vi "Setup TS.vi"(8 "error in":errorcluster, 11 "HTS Test Stand in":refnum<class "HTS Test Stand.lvclass">) -> (0 "error out":errorcluster, 3 "HTS Test Stand out":refnum<class "HTS Test Stand.lvclass">)   [LabVIEW 2019, in "Test Stands.lvlib" / "HTS Test Stand.lvclass"]
uses:
  HTS Test Stand.lvclass
  C:/Users/wg/Documents/LV_Projects/test-stand/App/Generic Test Stand/Generic Test Stand.lvclass
  DAC/HTS/Vacum Valve/DAC Vacum Valve.lvclass
  C:/Users/wg/Documents/LV_Projects/test-stand/App/DAC/DAC.lvclass
  DAC/HTS/Vacum Pressure/DAC Vacum Pressure.lvclass
  DAC/HTS/DC Supply/DAC DC Supply.lvclass
  DAC/HTS/LN2 Temp/DAC LN2 Temp.lvclass
  DAC/HTS/HTS dU/DAC HTS dU.lvclass
  DAC/DAC.lvclass/DAC.ctl
  Generic Test Stand/Generic Test Stand.lvclass/Generic Test Stand.ctl
  Generic Test Stand/Generic Test Stand.lvclass
  DAC/DAC.lvclass
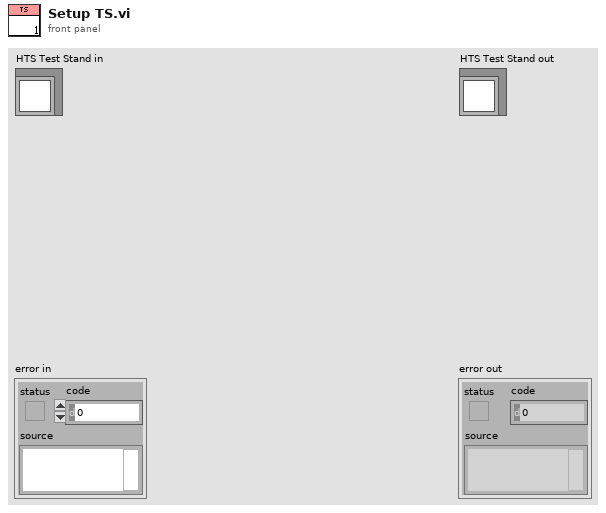
[diagram p1: front panel]
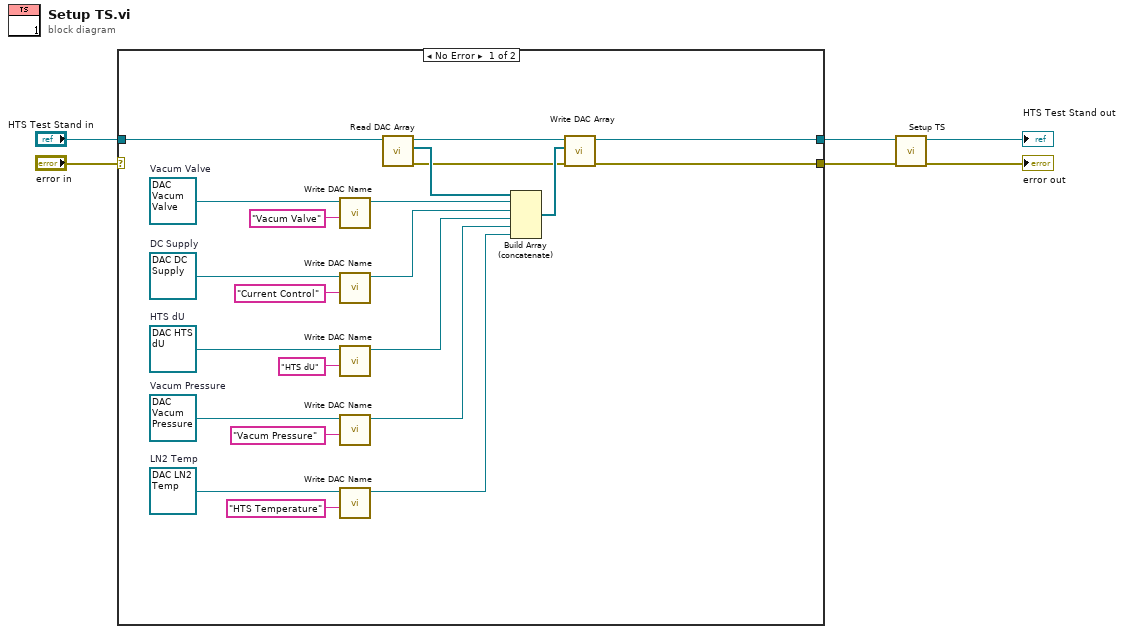
[diagram p0: block diagram]
diagram:
  n1 = case shown="No Error" "error in" {
    selector: "error in" -> [_ w29]
    tunnel: "HTS Test Stand in" -> [w28 w30]
    tunnel: [w22 w30] -> w2
    tunnel: [w21 w29] -> w1
    frame No Error {
      w11 = refnum<class "DAC HTS dU.lvclass"> refnum  # HTS dU
      w12 = refnum<class "DAC LN2 Temp.lvclass"> refnum  # LN2 Temp
      w13 = refnum<class "DAC DC Supply.lvclass"> refnum  # DC Supply
      w14 = refnum<class "DAC Vacum Pressure.lvclass"> refnum  # Vacum Pressure
      w15 = refnum<class "DAC Vacum Valve.lvclass"> refnum  # Vacum Valve
      n2 = call "Write DAC Name.vi"("DAC Name"="Vacum Valve", "DAC in"=w15) -> ("DAC out"=w23:refnum<class "DAC Vacum Valve.lvclass">)  [unwired: 8 in, 1 out]
      n3 = call "Write DAC Name.vi"("DAC Name"="Current Control", "DAC in"=w13) -> ("DAC out"=w10:refnum<class "DAC DC Supply.lvclass">)  [unwired: 8 in, 1 out]
      n4 = call "Write DAC Name.vi"("DAC Name"="HTS dU", "DAC in"=w11) -> ("DAC out"=w9:refnum<class "DAC HTS dU.lvclass">)  [unwired: 8 in, 1 out]
      n5 = call "Write DAC Name.vi"("DAC Name"="Vacum Pressure", "DAC in"=w14) -> ("DAC out"=w8:refnum<class "DAC Vacum Pressure.lvclass">)  [unwired: 8 in, 1 out]
      n6 = call "Write DAC Name.vi"("DAC Name"="HTS Temperature", "DAC in"=w12) -> ("DAC out"=w7:refnum<class "DAC LN2 Temp.lvclass">)  [unwired: 8 in, 1 out]
      n7 = call "Read DAC Array.vi"("Generic Test Stand in"=w28) -> ("error out"=w24:errorcluster, "DAC Array"=w27:refnum<class "DAC.lvclass">[], "Generic Test Stand out"=w26:refnum<class "HTS Test Stand.lvclass">)  [unwired: 8 in]
      n8 = Build Array (concatenate)(w27, w23, w10, w9, w8, w7) -> (w25:refnum<class "DAC.lvclass">[])
      n9 = call "Write DAC Array.vi"("error in (no error)"=w24, "DAC Array"=w25, "Generic Test Stand in"=w26) -> ("error out"=w21:errorcluster, "Generic Test Stand out"=w22:refnum<class "HTS Test Stand.lvclass">)  [unwired: 7 in]
    }
    frame Error {
    }
  }
  n10 = call-parent "Setup TS.vi"("error in (no error)"=w1, "Generic Test Stand in"=w2) -> ("error out"=→"error out":errorcluster, "Generic Test Stand out"=→"HTS Test Stand out":refnum<class "HTS Test Stand.lvclass">)  [unwired: 8 in]
